vi "Read Input Register Channels.vi"(8 "error in (no error)":errorcluster, 9 "Channels in":T1[](array[typedef]) {"Mapping"."VS Reference" format="%.0x"}, 11 "Modbus Master in":refnum<class "Modbus Master.lvclass">=refnum) -> (0 "error out":errorcluster, 2 "Input Registers out":dbl[](array[numeric]), 3 "Modbus Master out":refnum<class "Modbus Master.lvclass">)   [LabVIEW 2021]
uses:
  Modbus API.lvlibp/API/Master/Modbus Master.lvclass
  System Explorer/SubVIs/Modbus Type.ctl
  Shared/Modbus Master Shared.lvlib
  Shared/Controls/Data Model/Channel.ctl
  Shared/Controls/Data Model/DataType.ctl
  Shared/Controls/Data Model/Mapping.ctl
  <vilib>/NI VeriStand/Custom Device API/Custom Device Channel Type.ctl
  <vilib>/NI VeriStand/Custom Device API/Custom Device API.lvlib
  <vilib>/NI VeriStand/Custom Device API/Custom Device Item Ref.ctl
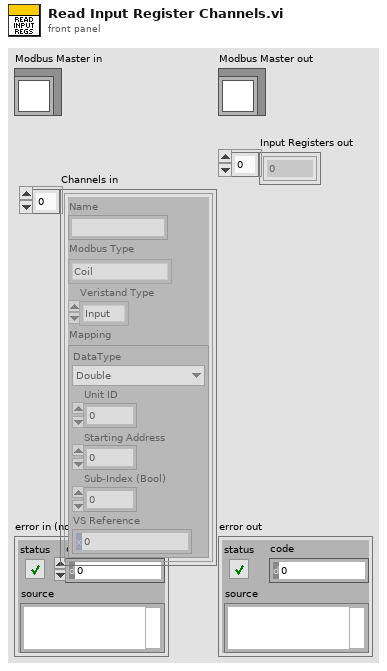
[diagram p1: front panel]
types:
  T1 = typedef "Modbus Master Shared.lvlib/Channel.ctl" = cluster{"Name":string, "Modbus Type":T2, "Veristand Type":T3, "Mapping":T4}
  T2 = typedef "Modbus Master Shared.lvlib/Modbus Type.ctl" = enum16{"Coil", "Discrete Input", "Holding Register", "Input Register"}
  T3 = typedef "Custom Device API.lvlib/Custom Device Channel Type.ctl" = enum16{"Input", "Output"}
  T4 = typedef "Modbus Master Shared.lvlib/Mapping.ctl" = cluster{"DataType":T5, "Unit ID":u8, "Starting Address":u16, "Sub-Index (Bool)":u16, "VS Reference":T6}
  T5 = typedef "Modbus Master Shared.lvlib/DataType.ctl" = enum16{"Double", "Single", "I64", "I32", "I16", "I8", "U64", "U32", "U16", "U8", "Boolean"}
  T6 = typedef "Custom Device API.lvlib/Custom Device Item Ref.ctl" = u64
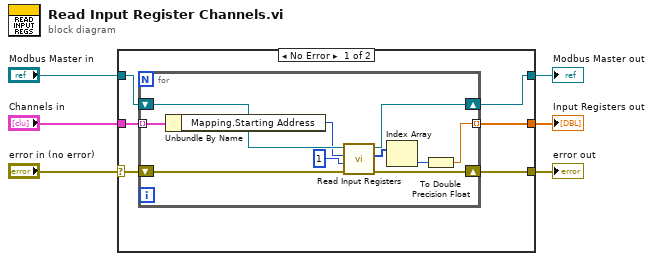
[diagram p0: block diagram]
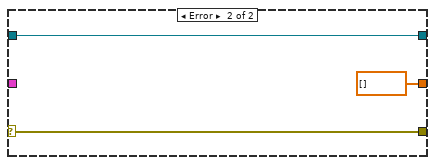
[diagram p2: hidden frame]
diagram:
  n1 = case shown="No Error" "error in (no error)" {
    selector: "error in (no error)" -> [w12 w23]
    tunnel: [w11 w24] -> w5
    tunnel: "Modbus Master in" -> [w10 w24]
    tunnel: [w9 w23] -> w3
    tunnel: "Channels in" -> [w8 _]
    tunnel: [w7 dbl[] []] -> w1
    frame No Error {
      n2 = for {
        shift-right: [w16] -> w9
        shift-left: w12 -> [w17]
        tunnel: w8 -> [w22] mode=indexing
        shift-right: [w20] -> w11
        shift-left: w10 -> [w21]
        tunnel: [w13] -> w7 mode=indexing
        n3 = Unbundle By Name(w22) -> ("Mapping.Starting Address"=w19:u16)
        n4 = call-dynamic "Read Input Registers.vi"("error in"=w17, "number of inputs"=u16 1, "starting address"=w19, "Modbus master in"=w21) -> ("error out"=w16:errorcluster, "register values"=w15:u16[], "Modbus master out"=w20:refnum<class "Modbus Master.lvclass">)  [unwired: 5 in]
        n5 = Index Array(array=w15) -> (element=w14:u16)  [unwired: 1 in]
        n6 = To Double Precision Float(number=w14) -> (double precision float=w13:dbl)
      }
    }
    frame Error {
    }
  }
  "Input Registers out" <- w1
  "Modbus Master out" <- w5
  "error out" <- w3
